vi "Initialise.vi"(8 "error in (no error)":errorcluster, 10 "Instrument Ref":string, 11 "Hioki BT4560B":refnum<class "Hioki BT4560B.lvclass">) -> (0 "error out":errorcluster, 3 "Hioki BT4560B":refnum<class "Hioki BT4560B.lvclass">)   [LabVIEW 2019, in "Concrete.lvlib" / "Hioki BT4560B.lvclass"]
uses:
  Hioki BT4560B.lvclass
  Hioki BT4560B.lvclass/Hioki BT4560B.ctl
  Harware Abstraction/Analog In/Analog In.lvclass
  <instrlib>/HIOKI BT4560/HIOKI BT4560.lvlib
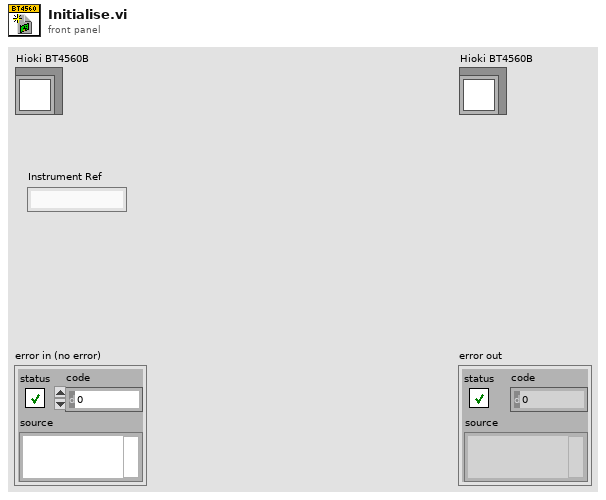
[diagram p1: front panel]
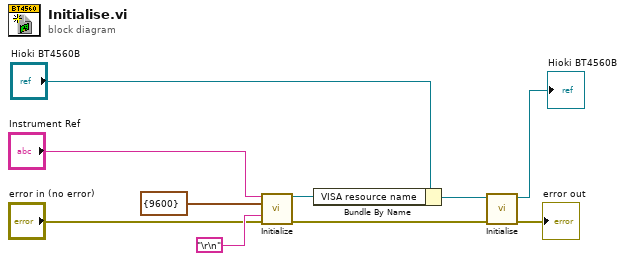
[diagram p0: block diagram]
diagram:
  n1 = call <instrlib>:"Initialize.vi"("VISA resource name"="Instrument Ref", "Serial Configuration"=cluster{"Baud Rate":u32} {"Baud Rate"=9600} ("Configuration"), "Terminator"="\r\n", "error in (no error)"="error in (no error)") -> ("VISA resource name out"=w3:refnum<visa-resource-name>, "error out"=w4:errorcluster)  [unwired: 9 in, 1 out]
  n2 = Bundle By Name(cluster="Hioki BT4560B", "VISA resource name"=w3) -> (w9:refnum<class "Hioki BT4560B.lvclass">)
  n3 = call-parent "Initialise.vi"("error in (no error)"=w4, "Instrument in"=w9) -> ("error out"=→"error out":errorcluster, "Instrument out"=→"Hioki BT4560B":refnum<class "Hioki BT4560B.lvclass">)  [unwired: 8 in]
